vi "Motor Power simple.vi"(9 "Motor":i16, 11 "data":waveform(dbl)[](array[waveform])) -> (1 "Power":waveform(dbl), 2 "Phase Current":waveform(dbl)(graph), 3 "Phase to Phase Voltage":waveform(dbl)(graph))   [LabVIEW 2011]
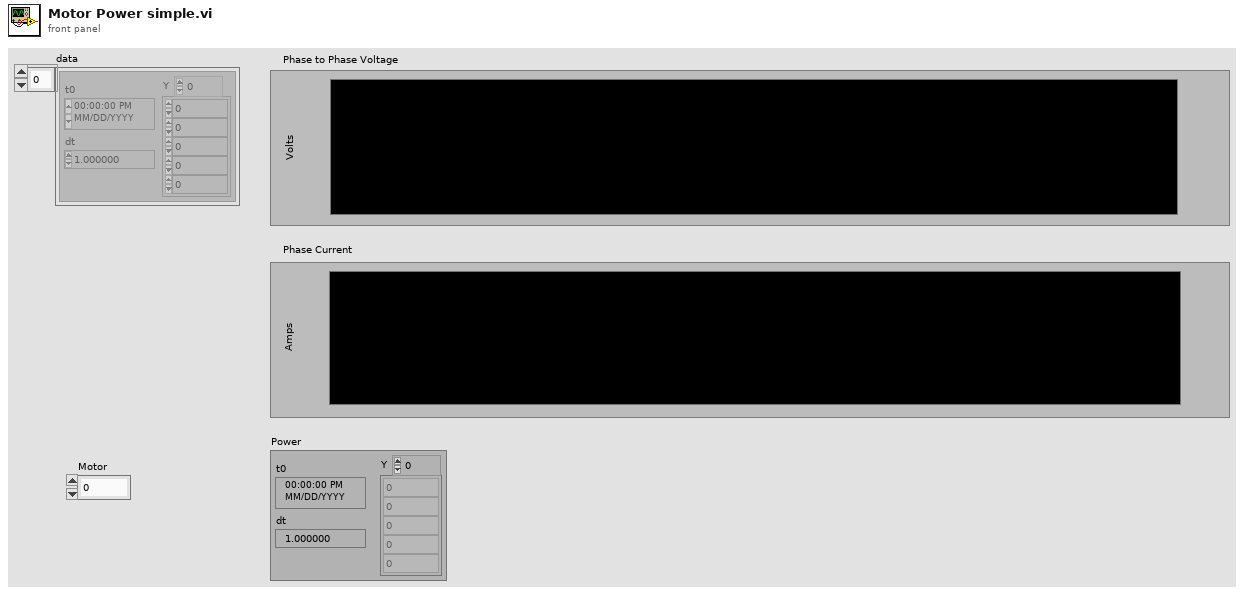
[diagram p1: front panel]
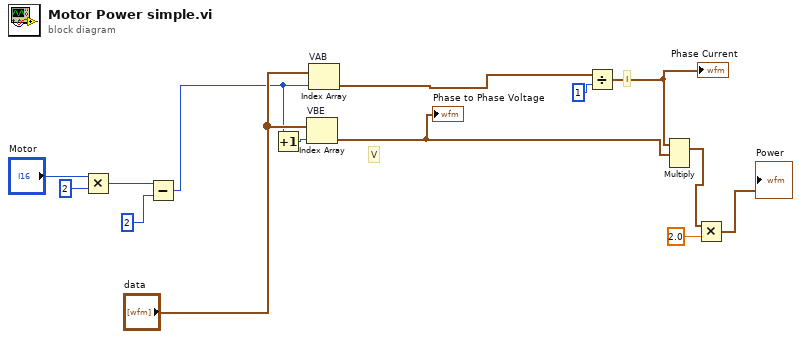
[diagram p0: block diagram]
diagram:
  # "I"
  # "V"
  n1 = Multiply(x="Motor", y=i16 2) -> (x*y=w5:i16)
  n2 = Subtract(x=w5, y=i16 2) -> (x-y=w6:i16)
  n3 = Increment(x=w6) -> (x+1=w7:i16)
  n4 = Index Array "VBE"(array="data", index=w7) -> (element=w14:waveform(dbl))
  "Phase to Phase Voltage" <- w14
  n5 = Index Array "VAB"(array="data", index=w6) -> (element=w13:waveform(dbl))
  n6 = Divide(x=w13, y=1) -> (x/y=w12:waveform(dbl))
  "Phase Current" <- w12
  n7 = Multiply(1:w14, 2:w12) -> (0:w3:waveform(dbl))  [unwired: 1 in, 1 out]
  n8 = Multiply(x=w3, y=2.0) -> (x*y=→"Power":waveform(dbl))
